vi "Panel.vi"(11 "Value Editor Base in":refnum<class "Value Editor Base.lvclass">) -> ()   [LabVIEW 2020, in "Value Editor Base.lvclass"]
uses:
  Value Editor Base.lvclass
  C:/Program Files (x86)/National Instruments/LabVIEW 2020/vi.lib/IlluminatedG/IG OOPanel/OOPanel/Panel/Panel.lvclass
  <vilib>/IlluminatedG/IG OOPanel/OOPanel/Panel/Basic UI State.ctl
  Value Editor Base.lvclass/Value Editor Base.ctl
  Special Terminal.ctl
  Value Mode.ctl
  Terminal Mode.ctl
  <vilib>/IlluminatedG/IG OOPanel/OOPanel/Panel/Panel.lvclass
  <vilib>/IlluminatedG/IG OOPanel/OOPanel/OOPanel.lvlib
  FlexBlocks.lvlib
panel:
  in  "Terminal Mode":T1(radio)=enum."Config"
  out "Supported Type":bool
  in  "Select Options":string(combo)
  out "Value Name":string
  out "Special Type":string
  in  "Value String":string
  out "Single Mode":string
  out "No Config Reason":string
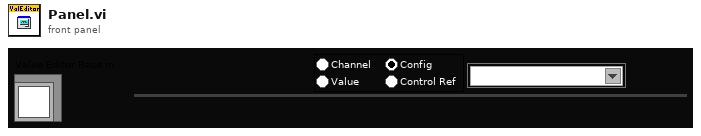
[diagram p1: front panel]
types:
  T1 = enum32{"Channel", "Config", "Value", "Control Ref"}
  T2 = typedef "OOPanel.lvlib/Panel.lvclass/Basic UI State.ctl" = enum16{"Init", "Run", "Close"}
  T3 = typedef "FlexBlocks.lvlib/Value Mode.ctl" = enum16{"Normal", "Range", "Select"}
  T4 = typedef "FlexBlocks.lvlib/Special Terminal.ctl" = enum16{"None", "Action", "Init", "Tag", "State in", "State out", "Error"}
  T5 = typedef "FlexBlocks.lvlib/Terminal Mode.ctl" = enum16{"Channel", "Config", "Value", "Control Ref"}
  T6 = typedef "Value Editor Base.lvclass/Inbound Events.ctl" = cluster{"Update Type":refnum<user-event>, "Update Terminal":refnum<user-event>, "Update Value":refnum<user-event>}
  T7 = typedef "OOPanel.lvlib/Panel.lvclass/Panel Events.ctl" = cluster{"Visbility":refnum<user-event>, "Close":refnum<user-event>}
  T8 = typedef "FlexBlocks.lvlib/Type Descriptor.ctl" = cluster{"Name":string, "Direction":T9, "Default":variant, "Min":variant, "Max":variant, "Step":variant, "Value Mode":T3, "Required":bool, "Connpane Index":i32, "Special Terminal":T4, "Color":u32, "Options":string[], "Type String":string, "Sort":i32, "Item Path":path}
  T9 = typedef "FlexBlocks.lvlib/Terminal Direction.ctl" = enum16{"Sink", "Source"}
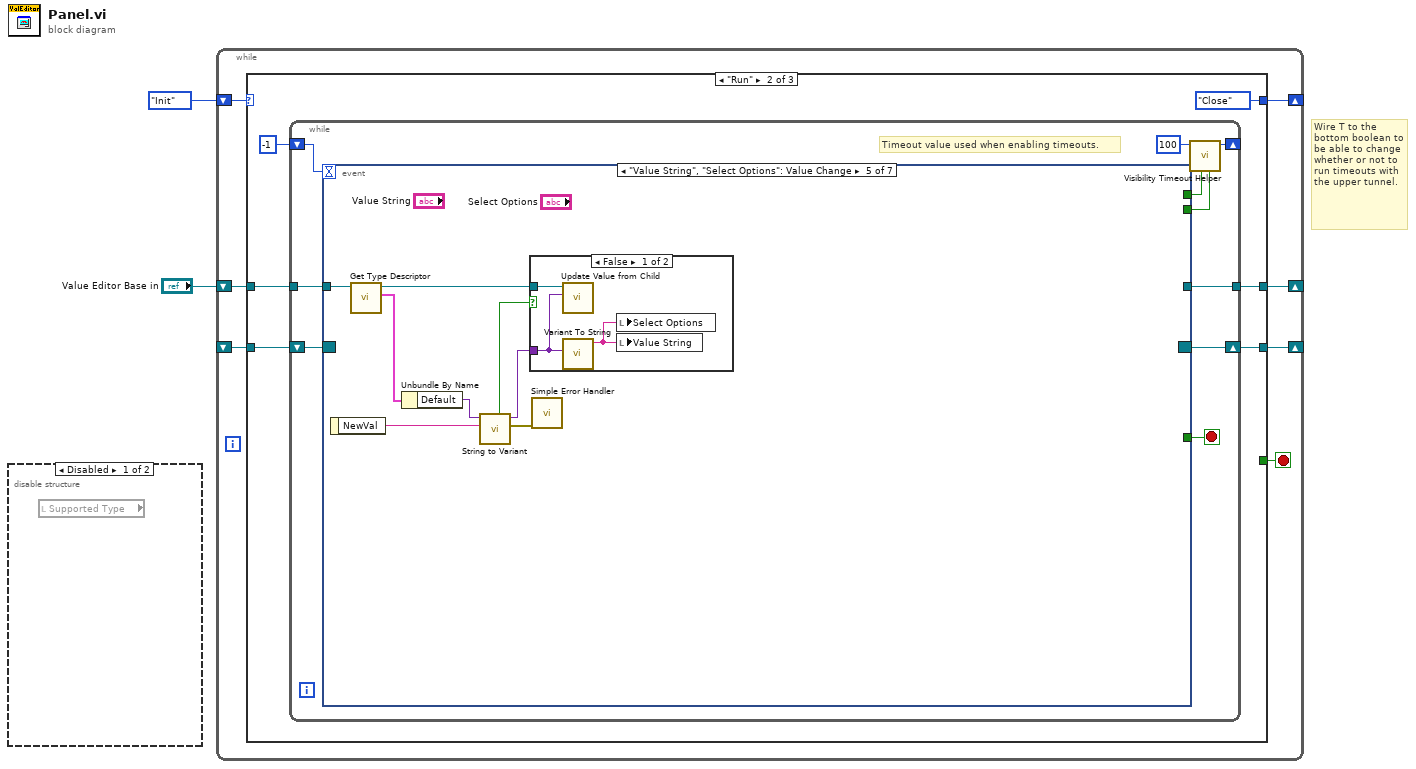
[diagram p0: block diagram]
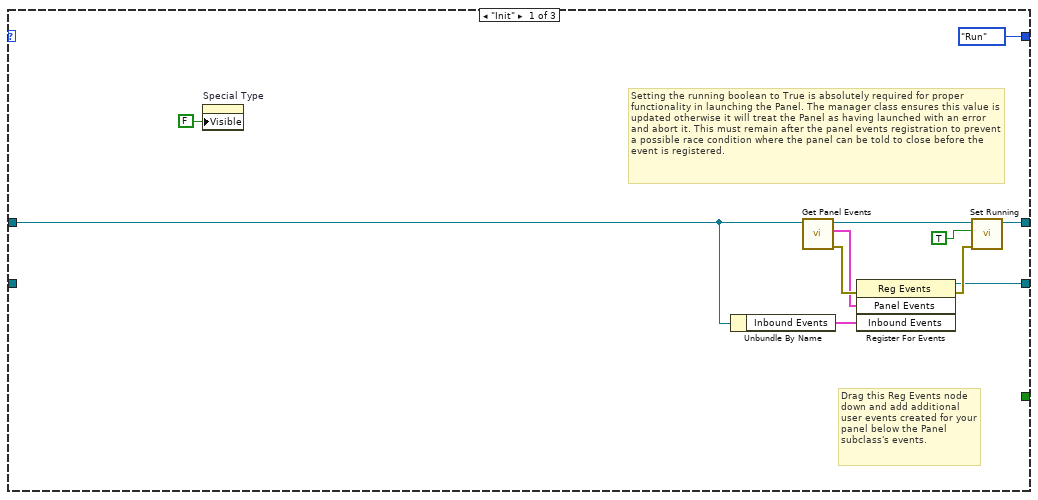
[diagram p3: hidden frame]
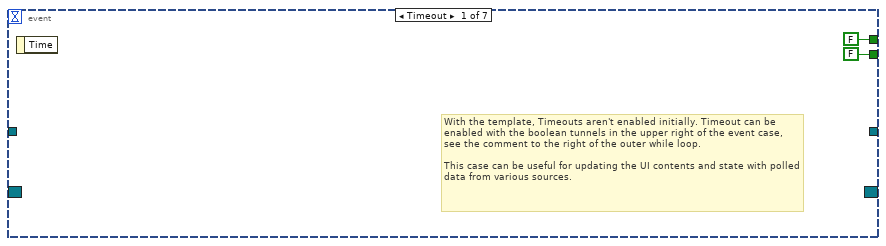
[diagram p4: hidden frame]
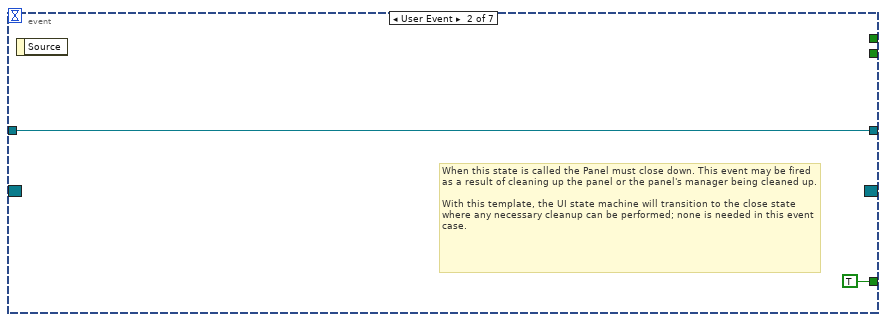
[diagram p5: hidden frame]
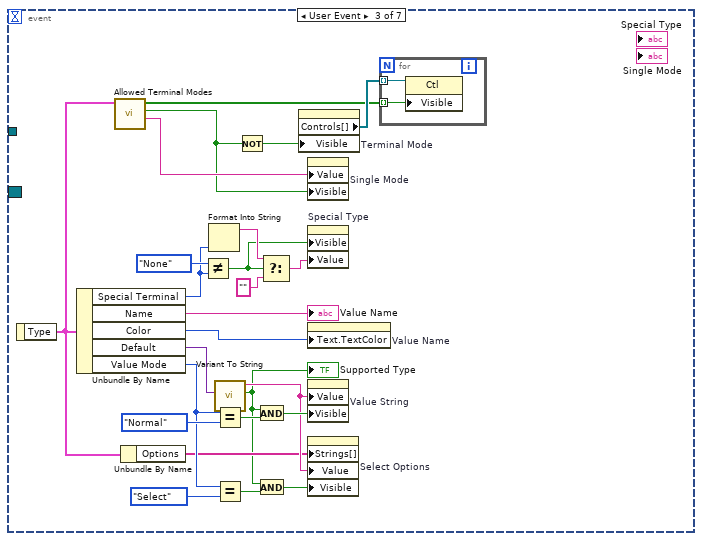
[diagram p6: hidden frame]
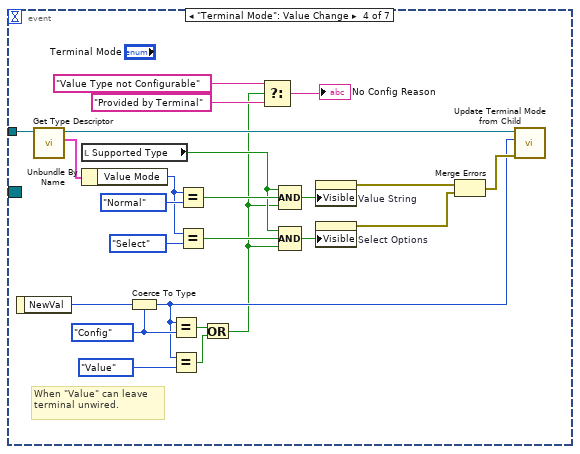
[diagram p7: hidden frame]
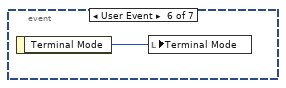
[diagram p9: hidden frame]
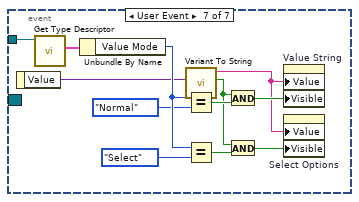
[diagram p10: hidden frame]
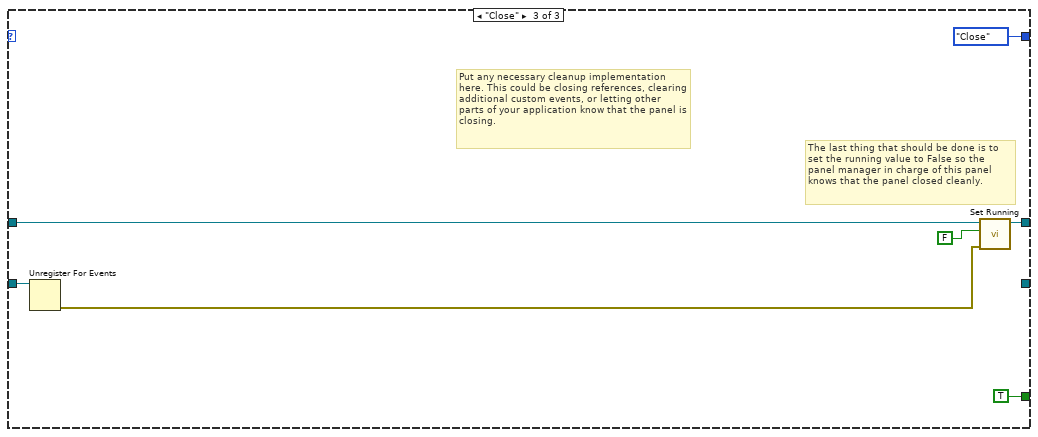
[diagram p11: hidden frame]
diagram:
  # "Wire T to the bottom boolean to be able to change whether or not to run timeouts with the upper tunnel."
  n1 = disable-structure shown="Disabled" {
    frame Disabled {
      n2 = local read "Supported Type"() -> ()  [unwired: 1 out]
    }
    frame Enabled {
    }
  }
  n3 = while {
    shift-right: [w8] -> _
    shift-left: _ -> [w9]
    shift-right: [w6] -> _
    shift-left: Basic_UI_State."Init" ("Basic UI State") -> [w7]
    shift-right: [w4] -> _
    shift-left: "Value Editor Base in" -> [w3]
    stop <- w5 stop-if-true
    n4 = case shown="\"Run\"" w7 {
      tunnel: w9 -> [_ w26 w118]
      tunnel: [w14 w24 _] -> w8
      tunnel: [Basic_UI_State."Run" ("Basic UI State") Basic_UI_State."Close" ("Basic UI State") Basic_UI_State."Close" ("Basic UI State")] -> w6
      tunnel: [_ _ TRUE] -> w5
      tunnel: [w13 w21 w116] -> w4
      tunnel: w3 -> [w12 w22 w117]
      frame "Init" {
        # "Setting the running boolean to True is absolutely required for proper functionality in launching the Panel. The manager class ensures this value is updated otherwise it will treat the Panel as having launched with an error and abort it. This must remain after the panel events registration to prevent a possible race condition where the panel can be told to close before the event is registered."
        # "Drag this Reg Events node down and add additional user events created for your panel below the Panel subclass's events."
        n5 = property on="Special Type" class="Str"("Visible"=FALSE) -> ()  [unwired: 2 in, 2 out]
        n6 = Unbundle By Name(w12) -> ("Inbound Events"=w11:T6)
        n7 = call <vilib>:"Get Panel Events.vi"("Panel in"=w12) -> ("error out"=w20:errorcluster, "Panel Events"=w16:T7, "Panel out"=w17:refnum<class "Value Editor Base.lvclass">)  [unwired: 8 in]
        n8 = register-events(error in=w20, w16, w11) -> (reference out=w14:refnum<event-registration>, error out=w18:errorcluster)  [unwired: 1 in]
        n9 = call <vilib>:"Set Running.vi"("error in (no error)"=w18, "Running"=TRUE, "Panel in"=w17) -> ("Panel out"=w13:refnum<class "Value Editor Base.lvclass">)  [unwired: 7 in, 1 out]
      }
      frame "Run" {
        n10 = while {
          shift-right: [w32] -> w24
          shift-left: w26 -> [w33]
          shift-right: [w35] -> _
          shift-left: -1 ("Timeout") -> [w34]
          tunnel: w22 -> [w28]
          tunnel: [w27] -> w21
          stop <- w29 stop-if-true
          # "Timeout value used when enabling timeouts."
          n11 = event shown="[4] \"Value String\", \"Select Options\": Value Change" {
            selector: w33 -> [_ _ _ _ _ _ _]
            dyn-events: [_ _ _ _ _ _ _] -> w32
            timeout: w34 -> [_ _ _ _ _ _ _]
            tunnel: [FALSE _ _ _ _ _ _] -> w31
            tunnel: [FALSE _ _ _ _ _ _] -> w30
            tunnel: [_ TRUE _ _ _ _ _] -> w29
            tunnel: w28 -> [_ w39 _ w87 w98 _ w115]
            tunnel: [_ w39 _ _ _ _ _] -> w27
            event Timeout {
              # "With the template, Timeouts aren't enabled initially. Timeout can be enabled with the boolean tunnels in the upper right of the event case, see the comment to the right of the outer while loop.\n\nThis case can be useful for updating the UI contents and state with polled data from various sources."
              n12 = event-data() -> ()  [unwired: 1 in, 1 out]
            }
            event User Event {
              # "When this state is called the Panel must close down. This event may be fired as a result of cleaning up the panel or the panel's manager being cleaned up.\n\nWith this template, the UI state machine will transition to the close state where any necessary cleanup can be performed; none is needed in this event case."
              n13 = event-data() -> ()  [unwired: 1 in, 1 out]
            }
            event User Event {
              n14 = event-data() -> ("Type"=w47:T8)  [unwired: 1 in]
              n15 = Unbundle By Name(w47) -> ("Special Terminal"=w62:T4, "Name"=→"Value Name":string, "Color"=w64:u32, "Default"=w55:variant, "Value Mode"=w52:T3)
              n16 = call "Allowed Terminal Modes.vi"("Type Descriptor"=w47) -> ("Single Mode String"=w46:string, "Single Mode?"=w45:bool, "Available Items"=w41:bool[])  [unwired: 8 in]
              n17 = Unbundle By Name(w47) -> ("Options"=w48:string[])
              n18 = Not Equal?(x=Special_Terminal."None", y=w62) -> (x != y?=w58:bool)
              n19 = Format Into String(w62) -> (resulting string=w61:string)  [unwired: 3 in, 1 out]
              n20 = call "Variant To String.vi"("Variant"=w55) -> ("Supported"=w44:bool, "String"=w49:string)  [unwired: 9 in]
              "Supported Type" <- w44
              n21 = Equal?(x=w52, y=Value_Mode."Normal") -> (x = y?=w56:bool)
              n22 = Equal?(x=w52, y=Value_Mode."Select") -> (x = y?=w51:bool)
              n23 = Not(x=w45) -> (.not. x?=w43:bool)
              n24 = And(x=w44, y=w56) -> (x .and. y?=w54:bool)
              n25 = And(x=w44, y=w51) -> (x .and. y?=w50:bool)
              n26 = Select(t=w61, s=w58, f="") -> (s? t:f=w59:string)
              n27 = property on="Terminal Mode" class="RadioBtnsControl (strict)"("Visible"=w43) -> ("Controls[]"=w42:refnum<vi>[])  [unwired: 2 in, 2 out]
              n28 = property on="Single Mode" class="Str"("Value"=w46, "Visible"=w45) -> ()  [unwired: 2 in, 2 out]
              n29 = property on="Special Type" class="Str"("Visible"=w58, "Value"=w59) -> ()  [unwired: 2 in, 2 out]
              n30 = property on="Value Name" class="Str"("Text.TextColor"=w64) -> ()  [unwired: 2 in, 2 out]
              n31 = property on="Value String" class="Str"("Value"=w49, "Visible"=w54) -> ()  [unwired: 2 in, 2 out]
              n32 = property on="Select Options" class="CmbBox"("Strings[]"=w48, "Value"=w49, "Visible"=w50) -> ()  [unwired: 2 in, 2 out]
              n33 = for {
                tunnel: w42 -> [w67] mode=indexing
                tunnel: w41 -> [w66] mode=indexing
                n34 = property class="Ctl"(reference=w67, "Visible"=w66) -> ()  [unwired: 1 in, 2 out]
              }
            }
            event "Terminal Mode": Value Change {
              w75 = Terminal_Mode."Config" ("y")
              # "When \"Value\" can leave terminal unwired."
              n35 = event-data() -> ("NewVal"=w76:T1)  [unwired: 1 in]
              n36 = call "Get Type Descriptor.vi"("Value Editor Base in"=w87) -> ("Type Descriptor"=w86:T8, "Value Editor Base out"=w77:refnum<class "Value Editor Base.lvclass">)  [unwired: 8 in, 1 out]
              n37 = local read "Supported Type"() -> (w80:bool)
              n38 = Unbundle By Name(w86) -> ("Value Mode"=w83:T3)
              n39 = Coerce To Type(0:w76, 1:w75) -> (2:w73:T5)
              n40 = Equal?(x=w73, y=w75) -> (x = y?=w72:bool)
              n41 = Equal?(x=w73, y=Terminal_Mode."Value") -> (x = y?=w71:bool)
              n42 = Equal?(x=w83, y=Value_Mode."Normal") -> (x = y?=w81:bool)
              n43 = Equal?(x=w83, y=Value_Mode."Select") -> (x = y?=w82:bool)
              n44 = Or(x=w72, y=w71) -> (x .or. y?=w70:bool)
              n45 = Select(t="Value Type not Configurable", s=w70, f="Provided by Terminal") -> (s? t:f=→"No Config Reason":string)
              n46 = Compound Arithmetic op=AND(w80, w81, w70) -> (w79:bool)
              n47 = Compound Arithmetic op=AND(w80, w82, w70) -> (w78:bool)
              n48 = property on="Value String" class="Str"("Visible"=w79) -> (error out=w69:errorcluster)  [unwired: 2 in, 1 out]
              n49 = property on="Select Options" class="CmbBox"("Visible"=w78) -> (error out=w68:errorcluster)  [unwired: 2 in, 1 out]
              n50 = Merge Errors(w69, w68) -> (w91:errorcluster)
              n51 = call "Update Terminal Mode from Child.vi"("error in (no error)"=w91, "Terminal Mode"=w73, "Value Editor Base in"=w77) -> ()  [unwired: 7 in, 2 out]
            }
            event "Value String", "Select Options": Value Change {
              n52 = event-data() -> ("NewVal"=w99:string)  [unwired: 1 in]
              n53 = call "Get Type Descriptor.vi"("Value Editor Base in"=w98) -> ("Type Descriptor"=w97:T8, "Value Editor Base out"=w93:refnum<class "Value Editor Base.lvclass">)  [unwired: 8 in, 1 out]
              n54 = Unbundle By Name(w97) -> ("Default"=w96:variant)
              n55 = call "String to Variant.vi"("String"=w99, "Type"=w96) -> ("error out"=w92:errorcluster, "Value"=w94:variant, "Invalid Format"=w95:bool)  [unwired: 7 in]
              n56 = case shown="False" w95 {
                tunnel: w94 -> [w101 _]
                tunnel: w93 -> [w102 _]
                frame False {
                  n57 = call "Update Value from Child.vi"("Value"=w101, "Value Editor Base in"=w102) -> ()  [unwired: 8 in, 2 out]
                  n58 = call "Variant To String.vi"("Variant"=w101) -> ("String"=w100:string)  [unwired: 9 in, 1 out]
                  n59 = local write "Select Options"(w100) -> ()
                  n60 = local write "Value String"(w100) -> ()
                }
                frame True {
                }
              }
              n61 = call <vilib>:"Simple Error Handler.vi"("error in (no error)"=w92) -> ()  [unwired: 4 in, 5 out]
            }
            event User Event {
              n62 = event-data() -> ("Terminal Mode"=w103:T5)  [unwired: 1 in]
              n63 = local write "Terminal Mode"(w103) -> ()
            }
            event User Event {
              n64 = event-data() -> ("Value"=w104:variant)  [unwired: 1 in]
              n65 = call "Get Type Descriptor.vi"("Value Editor Base in"=w115) -> ("Type Descriptor"=w114:T8)  [unwired: 8 in, 2 out]
              n66 = Unbundle By Name(w114) -> ("Value Mode"=w107:T3)
              n67 = call "Variant To String.vi"("Variant"=w104) -> ("Supported"=w109:bool, "String"=w108:string)  [unwired: 9 in]
              n68 = Equal?(x=w107, y=Value_Mode."Normal") -> (x = y?=w113:bool)
              n69 = Equal?(x=w107, y=Value_Mode."Select") -> (x = y?=w111:bool)
              n70 = And(x=w109, y=w113) -> (x .and. y?=w112:bool)
              n71 = And(x=w109, y=w111) -> (x .and. y?=w110:bool)
              n72 = property on="Value String" class="Str"("Value"=w108, "Visible"=w112) -> ()  [unwired: 2 in, 2 out]
              n73 = property on="Select Options" class="CmbBox"("Value"=w108, "Visible"=w110) -> ()  [unwired: 2 in, 2 out]
            }
          }
          n74 = call <vilib>:"Visibility Timeout Helper.vi"("Update?"=w30, "Use Timeout?"=w31, "Visible Timeout mS"=100) -> ("Timeout"=w35:i32)  [unwired: 8 in]
        }
      }
      frame "Close" {
        # "Put any necessary cleanup implementation here. This could be closing references, clearing additional custom events, or letting other parts of your application know that the panel is closing."
        # "The last thing that should be done is to set the running value to False so the panel manager in charge of this panel knows that the panel closed cleanly."
        n75 = Unregister For Events(event registration refnum=w118) -> (error out=w120:errorcluster)  [unwired: 1 in]
        n76 = call <vilib>:"Set Running.vi"("error in (no error)"=w120, "Running"=FALSE, "Panel in"=w117) -> ("Panel out"=w116:refnum<class "Value Editor Base.lvclass">)  [unwired: 7 in, 1 out]
      }
    }
  }
